vi "Device ID Ports.vi"(2 "Analysis Info cluster":T2[](array[typedef]) {"Kurt_u" format="%_3g"; "u^4" format="%_3g"; "u^3" format="%_3g"; "Sd Error in Variance" format="%_3g"; "u^2" format="%_3g"; "Sd Error in Mean" format="%_3g"; "U" format="%_3g"; "Sync Delay Time (s)" format="%.4f"; "Total Meas Time (s)" format="%_5g"; "Skew_u" format="%_3g"; "% u'/U" format="%_3g"}, 3 "DAQdeviceType":string) -> (0 "Unique Channel Names":string[](array[string]), 1 "Device port info":T1[](array[typedef]))   [LabVIEW 2022 SP3]
uses:
  Controls/Analysis_info_cluster.ctl
  Controls/Inst_type.ctl
  Controls/Instrument_Array.ctl
  Controls/channelState.ctl
  Device ID port info.ctl
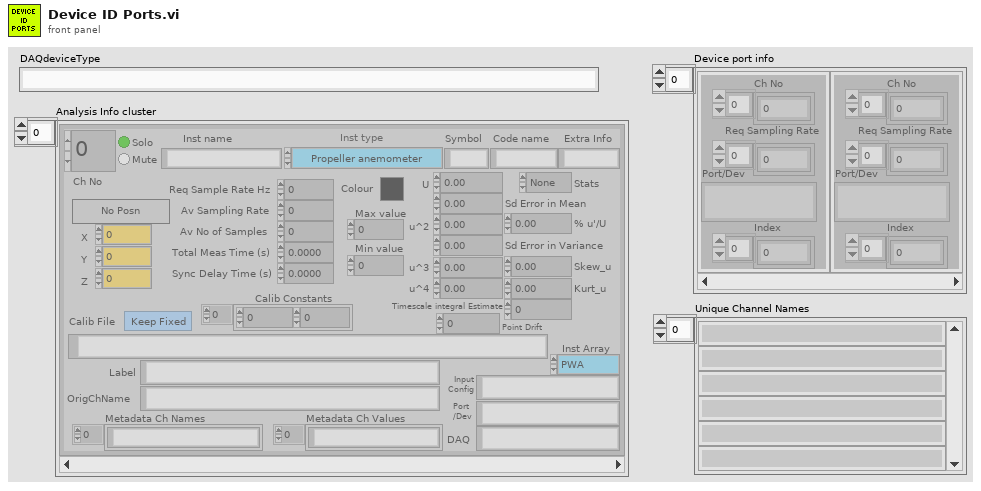
[diagram p1: front panel]
types:
  T1 = typedef "Device ID port info.ctl" = cluster{"Ch No":i16[], "Req Sampling Rate":dbl[], "Port":string, "Index":i32[]}
  T2 = typedef "Analysis_info_cluster.ctl" = cluster{"Colour":u32, "Inst type":T3, "Inst name":string, "Symbol":string, "Code name":string, "Extra Info":string, "Inst Array":T4, "U":dbl, "u^2":dbl, "u^3":dbl, "u^4":dbl, "Skew_u":dbl, "Kurt_u":dbl, "Sd Error in Mean":dbl, "% u'/U":dbl, "X":dbl, "Y":dbl, "Z":dbl, "Timescale integral Estimate":dbl, "Sd Error in Variance":dbl, "Calib File":path, "Calib Constants":dbl[], "Output Position":bool, "Stats":enum16{"None", "Basic", "Full"}, "Av Sampling Rate":dbl, "Av No of Samples":dbl, "Total Meas Time (s)":dbl, "OrigChName":string, "Max value":dbl, "Min value":dbl, "Req Sample Rate Hz":dbl, "Sync Delay Time (s)":dbl, "Ch No":i16, "Device":string, "Use Latest Calib":bool, "Port":string, "Metadata Ch Names":string[], "Metadata Ch Values":string[], "Label":string, "chState":T5, "Point Drift":dbl, "inputConfig":string}
  T3 = typedef "Inst_type.ctl" = enum16{"Raw voltage", "Raw with zero offsetting", "Propeller anemometer", "Pressure Transducer", "Pitot-static tube", "Hot wire", "Cross wire 1", "Cross wire 2", "Generic Linear", "Generic Polynomial", "Generic BackPoly", "Fast FID", "Thermocouple", "Cold wire", "Pulsed Wire", "LDA Vel", "LDA Tran time", "LDA Arr time", "Microphone"}
  T4 = typedef "Instrument_Array.ctl" = enum16{"PWA", "LDA", "Analogue"}
  T5 = typedef "channelState.ctl" = enum32{"No Selection", "Solo", "Mute"}
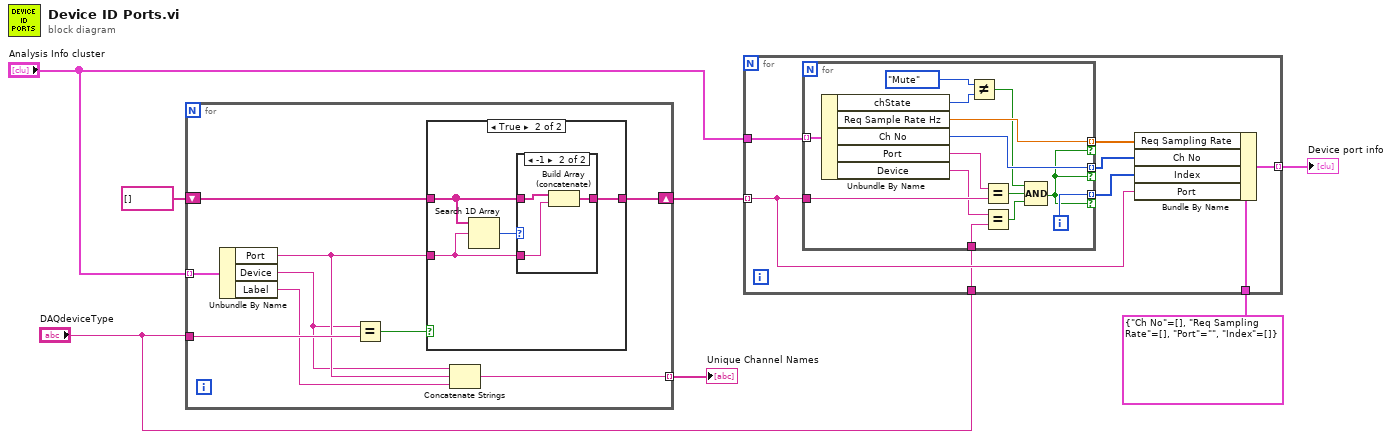
[diagram p0: block diagram]
diagram:
  n1 = for {
    tunnel: "Analysis Info cluster" -> [w14] mode=indexing
    shift-right: [w15] -> w5
    shift-left: string[] [] -> [w16]
    tunnel: [w13] -> w7 mode=indexing
    tunnel: "DAQdeviceType" -> [w12]
    n2 = Unbundle By Name(w14) -> ("Port"=w11:string, "Device"=w8:string, "Label"=w10:string)
    n3 = Equal?(x=w8, y=w12) -> (x = y?=w9:bool)
    n4 = case shown="True" w9 {
      tunnel: w16 -> [w17 w18]
      tunnel: w11 -> [_ w19]
      tunnel: [w17 w20] -> w15
      frame False {
      }
      frame True {
        n5 = Search 1D Array(1D array=w18, element=w19) -> (index of element=w21:i32)  [unwired: 1 in]
        n6 = case shown="-1" w21 {
          tunnel: w18 -> [w22 w25]
          tunnel: w19 -> [_ w24]
          tunnel: [w22 w23] -> w20
          frame Default {
          }
          frame -1 {
            n7 = Build Array (concatenate)(w25, w24) -> (w23:string[])
          }
        }
      }
    }
    n8 = Concatenate Strings(w8, w11, w10) -> (w13:string)
  }
  "Unique Channel Names" <- w7
  n9 = for {
    tunnel: w5 -> [w28] mode=indexing
    tunnel: "Analysis Info cluster" -> [w33]
    tunnel: T1 {"Ch No"=[], "Req Sampling Rate"=[], "Port"="", "Index"=[]} ("Cluster") -> [w32]
    tunnel: [w27] -> w2 mode=indexing
    tunnel: "DAQdeviceType" -> [w26]
    n10 = for {
      tunnel: w33 -> [w47] mode=indexing
      tunnel: w28 -> [w45]
      tunnel: [w44] -> w31 mode=indexing if=w38
      tunnel: [w43] -> w30 mode=indexing if=w38
      tunnel: [w42] -> w29 mode=indexing if=w38
      tunnel: w26 -> [w39]
      i -> [w42]
      n11 = Unbundle By Name(w47) -> ("chState"=w36:T5, "Req Sample Rate Hz"=w44:dbl, "Ch No"=w43:i16, "Port"=w46:string, "Device"=w40:string)
      n12 = Not Equal?(x=channelState."Mute" ("chState"), y=w36) -> (x != y?=w34:bool)
      n13 = Equal?(x=w46, y=w45) -> (x = y?=w41:bool)
      n14 = Equal?(x=w40, y=w39) -> (x = y?=w37:bool)
      n15 = Compound Arithmetic op=AND(w34, w41, w37) -> (w38:bool)
    }
    n16 = Bundle By Name(cluster=w32, "Req Sampling Rate"=w31, "Ch No"=w30, "Index"=w29, "Port"=w28) -> (w27:T1)
  }
  "Device port info" <- w2
